vi "CleanUp.vi"(5 "error in (no error)":errorcluster) -> (19 "error out":errorcluster)   [LabVIEW 2020, in "UmlEditor.lvclass"]
uses:
  <resource>/Framework/Providers/Open_GDS/UML/UmlEditor_class/UmlEditor.lvclass
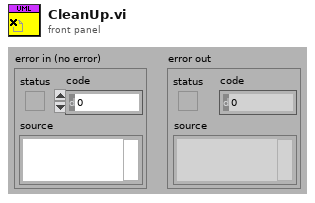
[diagram p1: front panel]
types:
  T1 = typedef "UmlEditor.lvclass/ObjectAttributes.ctl" = cluster{"ListeningQueueIn":refnum<queue>, "Event":refnum<user-event>, "UseProjectFolderAsBasePath":bool, "TypeSyncOption":bool, "Attr":string[], "ToolTip":cluster{"ToolTipOpen":bool, "LastToolTip":i32}, "ClassesToIgnore":string[], "UndoSize":i32, "OpenLastSavedFileWhenStarting":bool, "SyncOption":T2, "SyncTime(s)":i32, "Params":cluster{"IniParams":T3, "Value":string}[], "GraphButtons":refnum<vi>}
  T2 = typedef "UMLEditor_SyncOptions.ctl" = cluster{"IgnoreInstrLib":bool, "IgnoreUserLib":bool, "IgnoreViLib":bool}
  T3 = typedef "UmlEditor.lvclass/IniParamsType.ctl" = enum16{"I have problem with UML stability on my computer"}
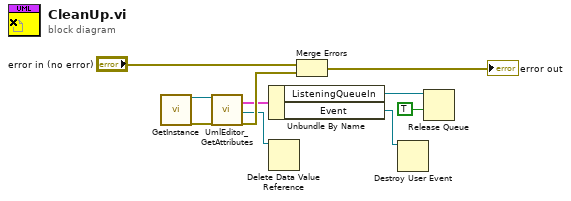
[diagram p0: block diagram]
diagram:
  n1 = call <resource>:"GetInstance.vi"() -> ("reference out"=w7:refnum<class "UmlEditor.lvclass">, "error out"=w6:errorcluster)  [unwired: 1 in, 17 out]
  n2 = call <resource>:"UmlEditor_GetAttributes.vi"("reference in"=w7, "error in (no error)"=w6) -> ("Data"=w2:T1, "DataRef"=w1:refnum<data-value>, "error out"=w8:errorcluster)  [unwired: 1 in, 14 out]
  n3 = Unbundle By Name(w2) -> ("ListeningQueueIn"=w5:refnum<queue>, "Event"=w3:refnum<user-event>)
  n4 = Delete Data Value Reference(data value reference=w1) -> ()  [unwired: 1 in, 2 out]
  n5 = Merge Errors("error in (no error)", w8) -> (→"error out":errorcluster)
  n6 = Destroy User Event(user event=w3) -> ()  [unwired: 1 in, 1 out]
  n7 = Release Queue(queue=w5, force destroy? (F)=TRUE) -> ()  [unwired: 1 in, 3 out]
